vi "MPM_Get_Sweep_Wavelength.vi"(8 "error in (no error)":errorcluster, 11 ".NET Reference in":refnum<k24>) -> (0 "error out":errorcluster, 1 "stopwave out":dbl, 2 "startwave out":dbl, 3 "Reference out":refnum<k24>, 5 "stepwave out":dbl)   [LabVIEW 2017]
uses:
  LV_IL_Sample/DLL/InstrumentDLL.dll
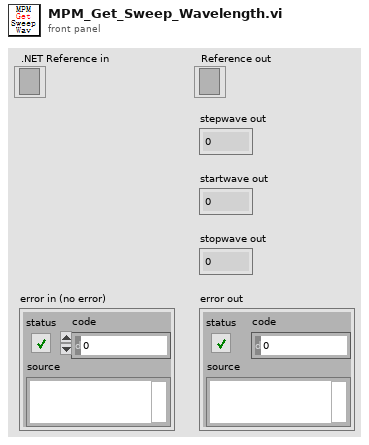
[diagram p1: front panel]
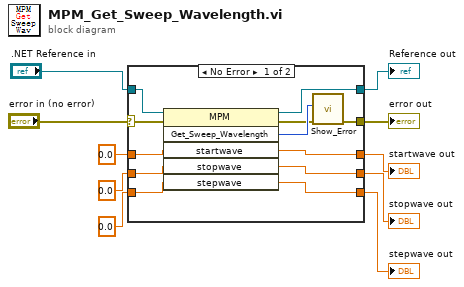
[diagram p0: block diagram]
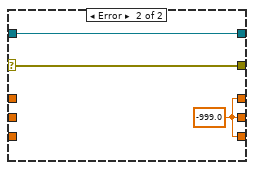
[diagram p2: hidden frame]
diagram:
  n1 = case shown="No Error" "error in (no error)" {
    selector: "error in (no error)" -> [w11 w25]
    tunnel: [w22 w24] -> w10
    tunnel: [w21 w23] -> w9
    tunnel: [w20 w23] -> w8
    tunnel: [w19 w23] -> w7
    tunnel: ".NET Reference in" -> [w18 w24]
    tunnel: 0.0 ("startwave") -> [w17 _]
    tunnel: 0.0 ("stopwave") -> [w16 _]
    tunnel: 0.0 ("stepwave") -> [w15 _]
    tunnel: [w12 w25] -> w2
    frame No Error {
      n2 = invoke class="MPM" method="Get_Sweep_Wavelength"(reference=w18, error in=w11, "startwave"=w17, "stopwave"=w16, "stepwave"=w15) -> (reference out=w22:refnum<k24>, error out=w13:errorcluster, "Get_Sweep_Wavelength"=w14:i32, "startwave"=w19:dbl, "stopwave"=w20:dbl, "stepwave"=w21:dbl)  [unwired: 1 in]
      n3 = call "Show_Error.vi"("error in (no error)"=w13, "Error"=w14) -> ("error out"=w12:errorcluster)  [unwired: 9 in]
    }
    frame Error {
      w23 = -999.0 ("startwave")
    }
  }
  "Reference out" <- w10
  "stepwave out" <- w9
  "stopwave out" <- w8
  "startwave out" <- w7
  "error out" <- w2
